vi "Get Variant Data Type.vi"(11 "variant":variant) -> (3 "Data Type":string[](array[string]))   [LabVIEW 2014]
doc: "Returns datatype as string from wired input. It tries to convert it to others datatypes and when it is possible it add this datatype into output list.\nSo if there is variant type i32 (32bit integer) it returns array ['double','i32'] because this value can be converted to double as well as to i32. solution is always take last array value."
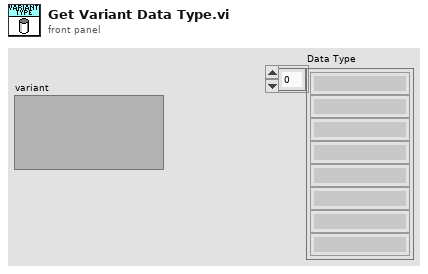
[diagram p1: front panel]
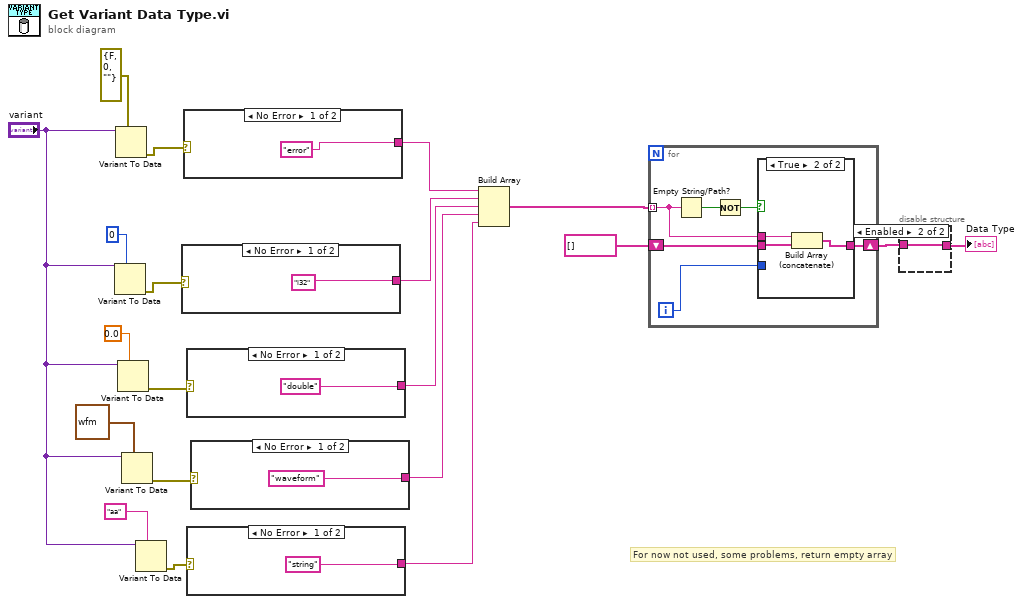
[diagram p0: block diagram]
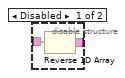
[diagram p2: hidden frame]
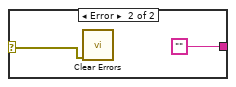
[diagram p4: hidden frame]
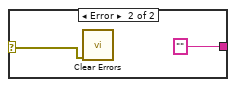
[diagram p5: hidden frame]
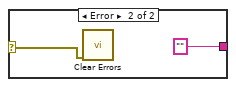
[diagram p6: hidden frame]
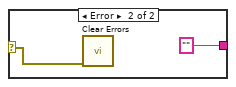
[diagram p7: hidden frame]
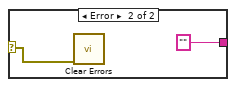
[diagram p8: hidden frame]
diagram:
  # "For now not used, some problems, return empty array"
  n1 = Variant To Data(type=0, Variant="variant") -> (error out=w17:errorcluster)  [unwired: 1 in, 1 out]
  n2 = Variant To Data(type=errorcluster {"status"=FALSE, "code"=0, "source"=""} ("error constant"), Variant="variant") -> (error out=w20:errorcluster)  [unwired: 1 in, 1 out]
  n3 = Variant To Data(type=0.0, Variant="variant") -> (error out=w15:errorcluster)  [unwired: 1 in, 1 out]
  n4 = Variant To Data(type=waveform(dbl) {"t0"=timestamp(0 s since 1904-01-01), "dt"=1.0, "Y"=[]} ("Waveform"), Variant="variant") -> (error out=w11:errorcluster)  [unwired: 1 in, 1 out]
  n5 = Variant To Data(type="aa" ("Data Type"), Variant="variant") -> (error out=w8:errorcluster)  [unwired: 1 in, 1 out]
  n6 = case shown="No Error" w17 {
    selector: w17 -> [_ w23]
    tunnel: ["i32" ("Data Type") "" ("Data Type")] -> w13
    frame No Error {
    }
    frame Error {
      n7 = call <vilib>:"Clear Errors.vi"("error in (no error)"=w23) -> ()  [unwired: 5 in, 2 out]
    }
  }
  n8 = case shown="No Error" w20 {
    selector: w20 -> [_ w26]
    tunnel: ["error" ("Data Type") "" ("Data Type")] -> w14
    frame No Error {
    }
    frame Error {
      n9 = call <vilib>:"Clear Errors.vi"("error in (no error)"=w26) -> ()  [unwired: 5 in, 2 out]
    }
  }
  n10 = case shown="No Error" w15 {
    selector: w15 -> [_ w29]
    tunnel: ["double" ("Data Type") "" ("Data Type")] -> w12
    frame No Error {
    }
    frame Error {
      n11 = call <vilib>:"Clear Errors.vi"("error in (no error)"=w29) -> ()  [unwired: 5 in, 2 out]
    }
  }
  n12 = case shown="No Error" w8 {
    selector: w8 -> [_ w32]
    tunnel: ["string" ("Data Type") "" ("Data Type")] -> w2
    frame No Error {
    }
    frame Error {
      n13 = call <vilib>:"Clear Errors.vi"("error in (no error)"=w32) -> ()  [unwired: 5 in, 2 out]
    }
  }
  n14 = case shown="No Error" w11 {
    selector: w11 -> [_ w35]
    tunnel: ["waveform" ("Data Type") "" ("Data Type")] -> w9
    frame No Error {
    }
    frame Error {
      n15 = call <vilib>:"Clear Errors.vi"("error in (no error)"=w35) -> ()  [unwired: 5 in, 2 out]
    }
  }
  n16 = Build Array(w14, w13, w12, w9, w2) -> (w5:string[])
  n17 = for {
    tunnel: w5 -> [w36] mode=indexing
    shift-right: [w38] -> w4
    shift-left: string[] [] ("appended array") -> [w40]
    i -> [w39]
    n18 = Empty String/Path?(string/path=w36) -> (empty?=w41:bool)
    n19 = Not(x=w41) -> (.not. x?=w37:bool)
    n20 = case shown="True" w37 {
      tunnel: w40 -> [w42 w45]
      tunnel: w39 -> [_ _]
      tunnel: [w42 w44] -> w38
      tunnel: w36 -> [_ w43]
      frame False {
      }
      frame True {
        n21 = Build Array (concatenate)(w43, w45) -> (w44:string[])
      }
    }
  }
  n22 = disable-structure shown="Enabled" {
    disable-tunnel: w4 -> [w47 w48]
    disable-tunnel: [w46 w48] -> w3
    frame Disabled {
      n23 = Reverse 1D Array(array=w47) -> (reversed array=w46:string[])
    }
    frame Enabled {
    }
  }
  "Data Type" <- w3
